vi "System Hidden.vi"(0 "Run Step Inputs":T2={"Data in"=[], "Results in"=[], "Seq Setup in"="", "Step name"="", "Hardware in"="", "Calibration in"="", "Step # in sequence"=0, "Display step?(f)"=TRUE, "Generate names only"=FALSE, "Waveforms in"=[], "Memory List Grouping info"=[]} {"Waveforms in"."Y dB ref" format="%.1f"; "Waveforms in"."Y axis" items=["dB", "Lin", "Pwr"]; "Waveforms in"."Y data" items=["dB", "Lin", "Pwr"]; "Waveforms in"."X data" items=["dB", "Lin", "Pwr"]; "Data in"."Z data" items=["dB", "Lin", "Pwr"]; "Data in"."X data" items=["dB", "Lin", "Pwr"]; "Data in"."Y data" items=["dB", "Lin", "Pwr"]; "Data in"."Z dB ref" format="%.1f"; "Data in"."Z axis" items=["Log", "Lin"]; "Data in"."X dB ref" format="%.1f"; "Data in"."X axis" items=["Log", "Lin"]; "Data in"."Y axis" items=["Log", "Lin"]; "Data in"."Y dB ref" format="%.1f"; "Data in"."Curve"."z" format="%.2f"; "Data in"."Curve"."y" format="%.2f"; "Data in"."Curve"."x" format="%.2f"; "Results in"."Unit type" items=["dB", "Lin", "Pwr"]; "Results in"."Margin" format="%.2f"}, 11 "error in (no error)":errorcluster) -> (6 "Data out":T3 {"Z data" items=["dB", "Lin", "Pwr"]; "X data" items=["dB", "Lin", "Pwr"]; "Y data" items=["dB", "Lin", "Pwr"]; "Z dB ref" format="%.1f"; "Z axis" items=["Log", "Lin"]; "X dB ref" format="%.1f"; "X axis" items=["Log", "Lin"]; "Y axis" items=["Log", "Lin"]; "Y dB ref" format="%.1f"; "Curve"."z" format="%.2f"; "Curve"."y" format="%.2f"; "Curve"."x" format="%.2f"}, 8 "Results out":T6 {"Unit type" items=["dB", "Lin", "Pwr"]; "Margin" format="%.2f"}, 10 "Waveforms out":T8 {"Y dB ref" format="%.1f"; "Y axis" items=["dB", "Lin", "Pwr"]; "Y data" items=["dB", "Lin", "Pwr"]; "X data" items=["dB", "Lin", "Pwr"]}, 15 "error out":errorcluster)   [LabVIEW 2016]
uses:
  custom and Sc run Seq Sub VIs (x64).llb/data array.ctl
  custom and Sc run Seq Sub VIs (x64).llb/data cluster.ctl
  custom and Sc run Seq Sub VIs (x64).llb/Axis Unit Type.ctl
  custom and Sc run Seq Sub VIs (x64).llb/result array.ctl
  custom and Sc run Seq Sub VIs (x64).llb/result cluster.ctl
  custom and Sc run Seq Sub VIs (x64).llb/waveform array.ctl
  custom and Sc run Seq Sub VIs (x64).llb/waveform cluster.ctl
  custom and Sc run Seq Sub VIs (x64).llb/Run Step Inputs.ctl
  custom and Sc run Seq Sub VIs (x64).llb/Memory List Grouping.ctl
  custom and Sc run Seq Sub VIs (x64).llb/Memory List Grouping - Item Type.ctl
  custom and Sc run Seq Sub VIs (x64).llb/memlist data type.ctl
panel:
  in  "custom setup cluster":T1={"Command Line"="", "Working Directory"=path "", "Wait for completion"=TRUE}
  # "NOTE:  These controls and indicators must stay here, but you can Hide them if you wish.  These are wired as the standard input/output connector pane for step run VIs."
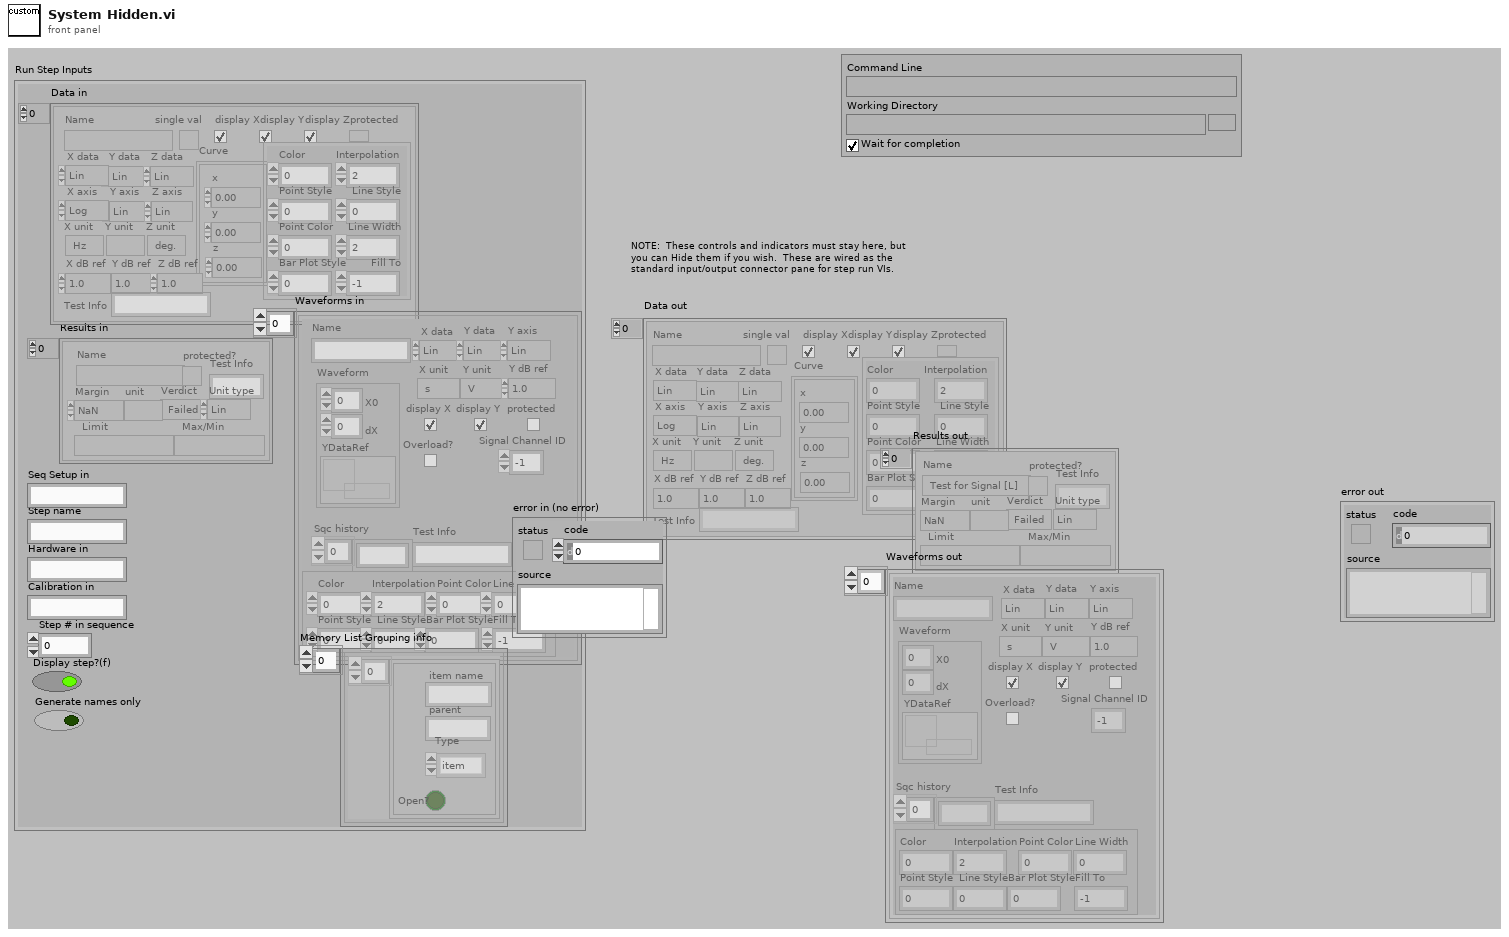
[diagram p1: front panel]
types:
  T1 = cluster{"Command Line":string, "Working Directory":path, "Wait for completion":bool}
  T2 = typedef "Run Step Inputs.ctl" = cluster{"Data in":T3, "Results in":T6, "Seq Setup in":string, "Step name":string, "Hardware in":string, "Calibration in":string, "Step # in sequence":i32, "Display step?(f)":bool, "Generate names only":bool, "Waveforms in":T8, "Memory List Grouping info":cluster{T10[]}[]}
  T3 = typedef "data array.ctl" = T4[]
  T4 = typedef "data cluster.ctl" = cluster{"Name":string, "Curve":cluster{"x":dbl, "y":dbl, "z":dbl}[], "X data":T5, "Y data":T5, "Z data":T5, "X axis":u16, "Y axis":u16, "Z axis":u16, "X unit":string, "Y unit":string, "Z unit":string, "X dB ref":dbl, "Y dB ref":dbl, "Z dB ref":dbl, "single val":bool, "protected":bool, "display X":bool, "display Y":bool, "display Z":bool, "Plot Settings":cluster{"Color":u32, "Interpolation":u8, "Point Style":u8, "Line Style":u8, "Point Color":u32, "Line Width":u8, "Bar Plot Style":u8, "Fill To":i16}, "Test Info":string}
  T5 = typedef "Axis Unit Type.ctl" = u16
  T6 = typedef "result array.ctl" = T7[]
  T7 = typedef "result cluster.ctl" = cluster{"Name":string, "Margin":dbl, "unit":string, "Verdict":bool, "Limit":string, "Max/Min":string, "protected?":bool, "Test Info":string, "Unit type":T5}
  T8 = typedef "waveform array.ctl" = T9[]
  T9 = typedef "waveform cluster.ctl" = cluster{"Name":string, "Waveform":cluster{"X0":dbl, "dX":dbl, "YDataRef":refnum<data-value>}, "X data":T5, "Y data":T5, "Y axis":T5, "X unit":string, "Y unit":string, "Y dB ref":dbl, "display Y":bool, "display X":bool, "Overload?":bool, "protected":bool, "Sqc history":string[], "Signal Channel ID":i32, "Plot Settings":cluster{"Color":u32, "Interpolation":u8, "Point Style":u8, "Line Style":u8, "Point Color":u32, "Line Width":u8, "Bar Plot Style":u8, "Fill To":i16}, "Test Info":string}
  T10 = typedef "Memory List Grouping.ctl" = cluster{"item name":string, "parent":string, "Open?":bool, "Type":T11}
  T11 = typedef "Memory List Grouping - Item Type.ctl" = enum16{"item", "custom group", "auto group", "protected group"}
  T12 = typedef "memlist data type.ctl" = enum32{"curve", "value", "result", "waveform"}
  T13 = typedef "seq step setup.ctl" = cluster{"Input Signal Channels":i32[], "Output Signal Channels":i32[], "Curves selected":string[][], "Curves generated":string[], "Step setup flat":string, "Trigger Signal Channel":i32, "Curves Generated Assumptions":cluster{"seq-setup in":string, "Relevant subset of mem list Grouping":cluster{T10[]}[]}}
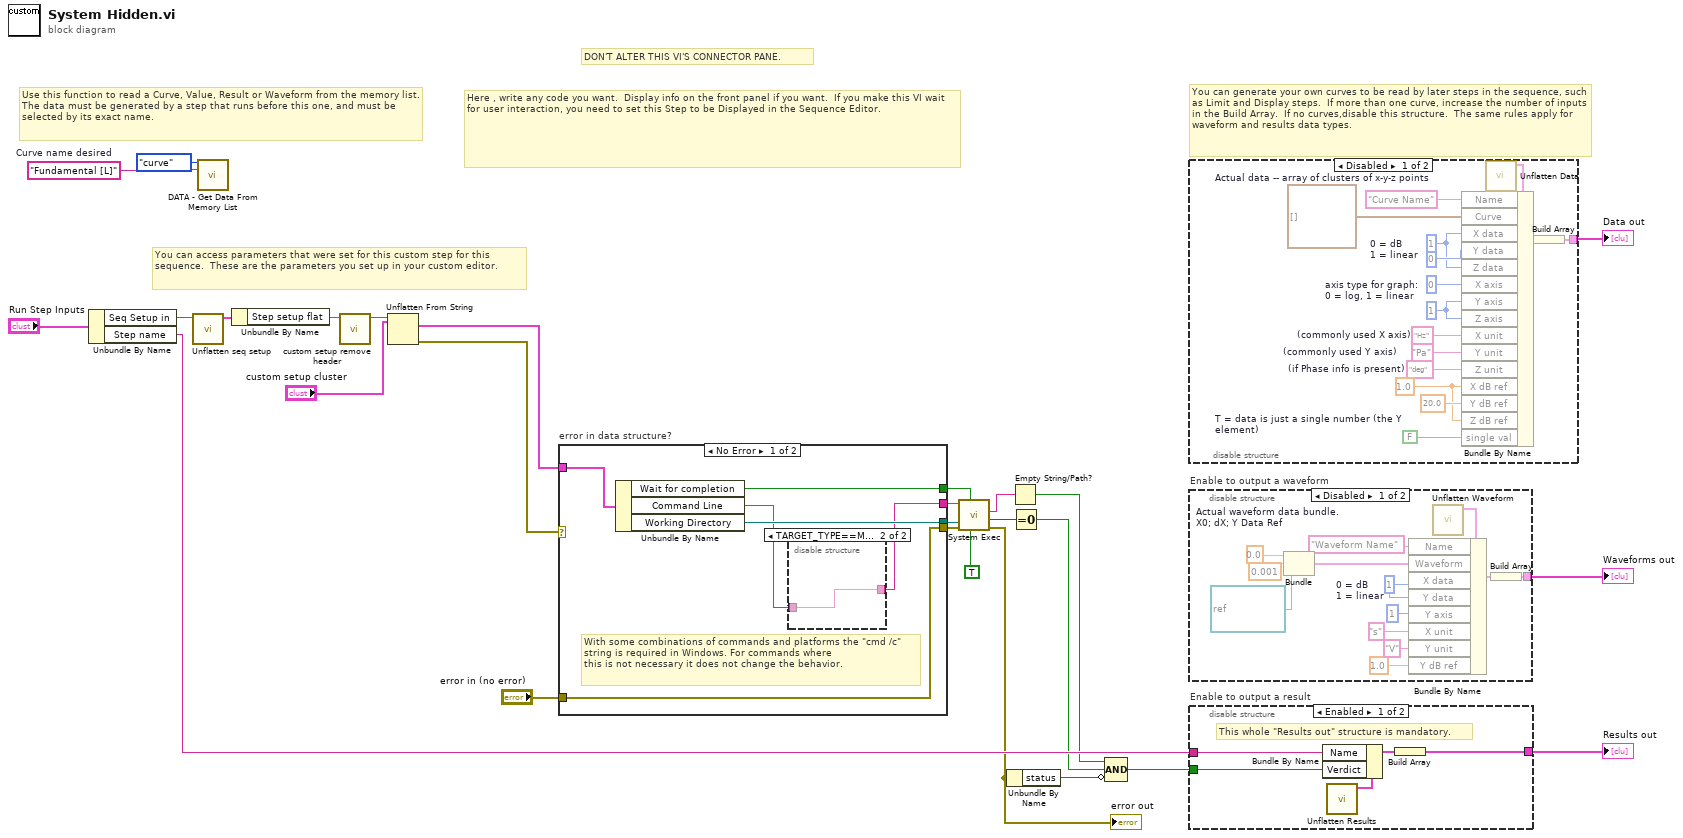
[diagram p0: block diagram]
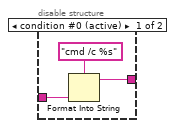
[diagram p2: hidden frame]
diagram:
  w18 = "Fundamental [L]"  # Curve name desired
  # "You can generate your own curves to be read by later steps in the sequence, such as Limit and Display steps.  If more than one curve, increase the number of inputs in the Build Array.  If no curves,disable this structure.  The same rules apply for waveform and results data types."
  # "Here , write any code you want.  Display info on the front panel if you want.  If you make this VI wait for user interaction, you need to set this Step to be Displayed in the Sequence Editor."
  # "Use this function to read a Curve, Value, Result or Waveform from the memory list. The data must be generated by a step that runs before this one, and must be selected by its exact name."
  # "You can access parameters that were set for this custom step for this sequence.  These are the parameters you set up in your custom editor."
  # "DON'T ALTER THIS VI'S CONNECTOR PANE."
  n1 = Unbundle By Name("Run Step Inputs") -> ("Seq Setup in"=w26:string, "Step name"=w15:string)
  n2 = call "Unflatten seq setup.vi"("Unflatten seq setup"=w26) -> ("Sequence-specific step set-up"=w25:T13)  [unwired: 3 in, 7 out]
  n3 = call "DATA - Get Data From Memory List.vi"("Data type"=memlist_data_type."curve", "Data Name"=w18) -> ()  [unwired: 7 in, 7 out]
  n4 = Unbundle By Name(w25) -> ("Step setup flat"=w24:string)
  n5 = call "custom setup remove header.vi"("Output from 'Step setup flat' of seq-setup structure"=w24) -> ("Flattened custom step setup cluster"=w23:string)  [unwired: 10 out]
  n6 = Unflatten From String(type="custom setup cluster", binary string=w23) -> (value=w12:T1, error out=w8:errorcluster)  [unwired: 1 in, 3 out]
  n7 = case "error in data structure?" shown="No Error" w8 {
    selector: w8 -> [_ w38]
    tunnel: [w29 _] -> w5
    tunnel: [w33 _] -> w16
    tunnel: w12 -> [w32 _]
    tunnel: [w31 _] -> w17
    tunnel: [w28 w38] -> w7
    tunnel: "error in (no error)" -> [w28 _]
    frame No Error {
      # "With some combinations of commands and platforms the \"cmd /c\" string is required in Windows. For commands where\nthis is not necessary it does not change the behavior."
      n8 = Unbundle By Name(w32) -> ("Wait for completion"=w31:bool, "Command Line"=w30:string, "Working Directory"=w33:path)
      n9 = disable-structure shown="TARGET_TYPE==Mac" {
        disable-tunnel: w30 -> [w36 w37]
        disable-tunnel: [w35 w37] -> w29
        frame condition #0 (active) {
          n10 = Format Into String(format string="cmd /c %s", w36) -> (resulting string=w35:string)  [unwired: 2 in, 1 out]
        }
        frame condition #1 {
        }
      }
    }
    frame Error {
    }
  }
  n11 = call <vilib>:"System Exec.vi"("run minimized? (F)"=TRUE, "wait until completion? (T)"=w17, "error in (no error)"=w7, "working directory"=w16, "command line"=w5) -> ("error out"=w14:errorcluster, "return code"=w3:i32, "standard error"=w4:string)  [unwired: 1 in, 3 out]
  "error out" <- w14
  n12 = Unbundle By Name(w14) -> ("status"=w11:bool)
  n13 = Empty String/Path?(string/path=w4) -> (empty?=w9:bool)
  n14 = Equal To 0?(x=w3) -> (x = 0?=w10:bool)
  n15 = Compound Arithmetic op=AND(w9, w10, invert w11) -> (w2:bool)
  n16 = disable-structure shown="Disabled" {
    disable-tunnel: [w53 _] -> w22
    frame Disabled {
      w51 = FALSE  # T = data is just a single number (the Y element)
      w49 = 1.0
      w46 = u16 1 ("Bundle Element")
      w48 = "deg"  # (if Phase info is present)
      w42 = "Hz"  # (commonly used X axis)
      w47 = "Pa"  # (commonly used Y axis)
      w45 = u16 0  # axis type for graph: 0 = log, 1 = linear
      w43 = u16 1  # 0 = dB 1 = linear
      w41 = cluster{"x":dbl, "y":dbl, "z":dbl}[] []  # Actual data -- array of clusters of x-y-z points
      n17 = call "Unflatten Data.vi"() -> ("Datum"=w39:T4)  [unwired: 1 in, 10 out]
      n18 = Bundle By Name(cluster=w39, "Name"="Curve Name" ("Bundle Element"), "Curve"=w41, "X data"=w43, "Y data"=u16 0 ("Bundle Element"), "Z data"=w43, "X axis"=w45, "Y axis"=w46, "Z axis"=w46, "X unit"=w42, "Y unit"=w47, "Z unit"=w48, "X dB ref"=w49, "Y dB ref"=20.0, "Z dB ref"=w49, "single val"=w51) -> (w52:T4)
      n19 = Build Array(w52) -> (w53:T4[])
    }
    frame Enabled {
    }
  }
  "Data out" <- w22
  n20 = disable-structure "Enable to output a waveform" shown="Disabled" {
    disable-tunnel: [w60 _] -> w21
    frame Disabled {
      w61 = u16 1  # 0 = dB 1 = linear
      n21 = Bundle "Actual waveform data bundle.\nX0; dX; Y Data Ref"(0.0, 0.001, "YDataRef"=refnum<data-value> refnum) -> (w54:cluster{dbl, dbl, "YDataRef":refnum<data-value>})  [unwired: 1 out]
      n22 = call "Unflatten Waveform.vi"() -> ("Unflattened Waveform"=w58:T9)  [unwired: 2 in, 9 out]
      n23 = Bundle By Name(cluster=w58, "Name"="Waveform Name" ("Bundle Element"), "Waveform"=w54, "X data"=w61, "Y data"=w61, "Y axis"=u16 1, "X unit"="s", "Y unit"="V", "Y dB ref"=1.0) -> (w59:T9)
      n24 = Build Array(w59) -> (w60:T9[])
    }
    frame Enabled {
    }
  }
  "Waveforms out" <- w21
  n25 = disable-structure "Enable to output a result" shown="Enabled" {
    disable-tunnel: [w71 _] -> w20
    disable-tunnel: w15 -> [w68 _]
    disable-tunnel: w2 -> [w67 _]
    frame Enabled {
      # "This whole \"Results out\" structure is mandatory."
      n26 = call "Unflatten Results.vi"() -> ("Result"=w69:T7)  [unwired: 1 in, 10 out]
      n27 = Bundle By Name(cluster=w69, "Name"=w68, "Verdict"=w67) -> (w70:T7)
      n28 = Build Array(w70) -> (w71:T7[])
    }
    frame Disabled {
    }
  }
  "Results out" <- w20
